vi "CSC_SetCuffs.vi"(8 "error in (no error)":errorcluster, 10 "Cuffs":T1[](array[typedef]), 11 "CableSerialChain in":refnum<class "CableSerialChain.lvclass">) -> (0 "error out":errorcluster, 3 "CableSerialChain out":refnum<class "CableSerialChain.lvclass">)   [LabVIEW 2015, in "CableSerialChain.lvclass"]
uses:
  CableSerialChain.lvclass
  TypeDef/Cuff.ctl
  Body/PointOnBody.ctl
  <vilib>/Analysis/Matrix/Datatypes/RealMatrix.ctl
  CableSerialChain.lvclass/CableSerialChain.ctl
  Body/Bodies.lvclass
  <vilib>/Analysis/Matrix/NI_Matrix.lvlib
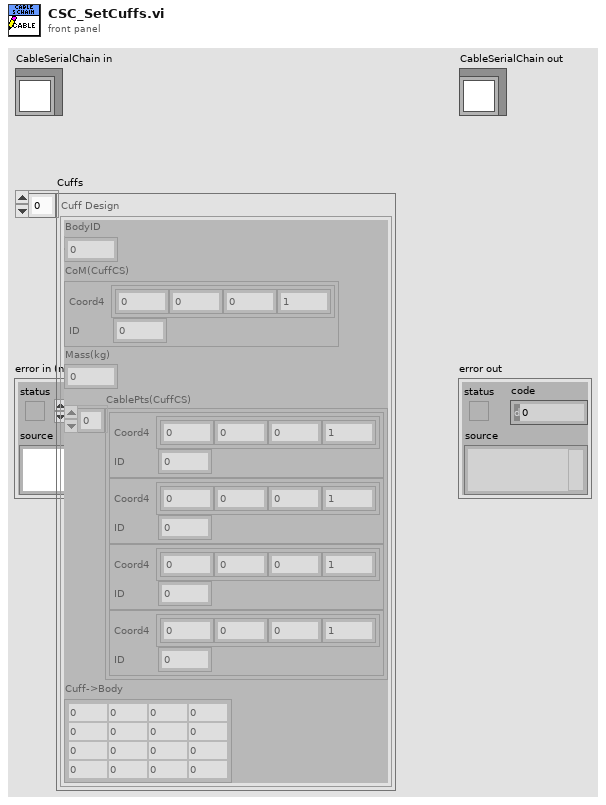
[diagram p1: front panel]
types:
  T1 = typedef "CableSerialChain.lvclass/Cuff.ctl" = cluster{"BodyID":i32, "CoM(CuffCS)":T2, "Mass(kg)":dbl, "CablePts(CuffCS)":T2[], "Cuff->Body":T3}
  T2 = typedef "Bodies.lvclass/PointOnBody.ctl" = cluster{"Coord4":dbl[], "ID":i32}
  T3 = typedef "NI_Matrix.lvlib/RealMatrix.ctl" = dbl[][]
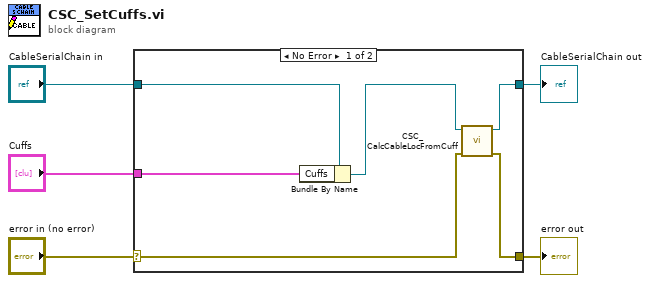
[diagram p0: block diagram]
diagram:
  n1 = case shown="No Error" "error in (no error)" {
    selector: "error in (no error)" -> [w7 w12]
    tunnel: [w6 w12] -> w4
    tunnel: [w8 w13] -> w2
    tunnel: "CableSerialChain in" -> [w11 w13]
    tunnel: "Cuffs" -> [w10 _]
    frame No Error {
      n2 = Bundle By Name(cluster=w11, "Cuffs"=w10) -> (w9:refnum<class "CableSerialChain.lvclass">)
      n3 = call "CSC_CalcCableLocFromCuff.vi"("error in (no error)"=w7, "C-Alex"=w9) -> ("error out"=w6:errorcluster, "C-Alex Out"=w8:refnum<class "CableSerialChain.lvclass">)  [unwired: 8 in]
    }
    frame Error {
    }
  }
  "error out" <- w4
  "CableSerialChain out" <- w2
